vi "读取excel数据并分析.vi"() -> ()   [LabVIEW 2012]
uses:
  <vilib>/Utility/NIReport.llb/NI_report.lvclass
  <vilib>/addons/_office/excel.llb/Excel Get Data ([str]).vi
  <vilib>/addons/_office/excel.llb/Excel Easy Table (str).vi
  <vilib>/Utility/NIReport.llb/Excel/NI_Excel.lvclass
  <vilib>/addons/_office/NI_ReportGenerationToolkit.lvlib
  <vilib>/Analysis/NI_AALPro.lvlib
panel:
  in  "数据量（随具体量修改）":i32=160
  out "数组":dbl[][](array[numeric])
  out "F-格式字符串":string[][](array[string])
  in  "写入start (0, 0) 2":cluster{"row":i32, "column":i32}
  out "error out 2":errorcluster caption="错误输出"
  in  "worksheet index (0) 2":i32
  in  "template (empty) 2":path caption="写入文件位置"
  in  "error in (no error) 2":errorcluster caption="错误输入（无错误）"
  out "截距":dbl[](array[numeric])
  out "斜率":dbl[](array[numeric])
  out "子数组":dbl[](array[numeric])
  in  "读出end (-1, -1)":cluster{"row":i32, "column":i32}={"row"=-1, "column"=-1}
  out "data":string[][](array[string])
  in  "读出start (0, 0)":cluster{"start row":i32, "start column":i32}
  in  "worksheet index (0)":i32
  in  "template (empty)":path caption="读取文件位置"
  in  "error in (no error)":errorcluster caption="错误输入（无错误）"
  out "error out":errorcluster caption="错误输出"
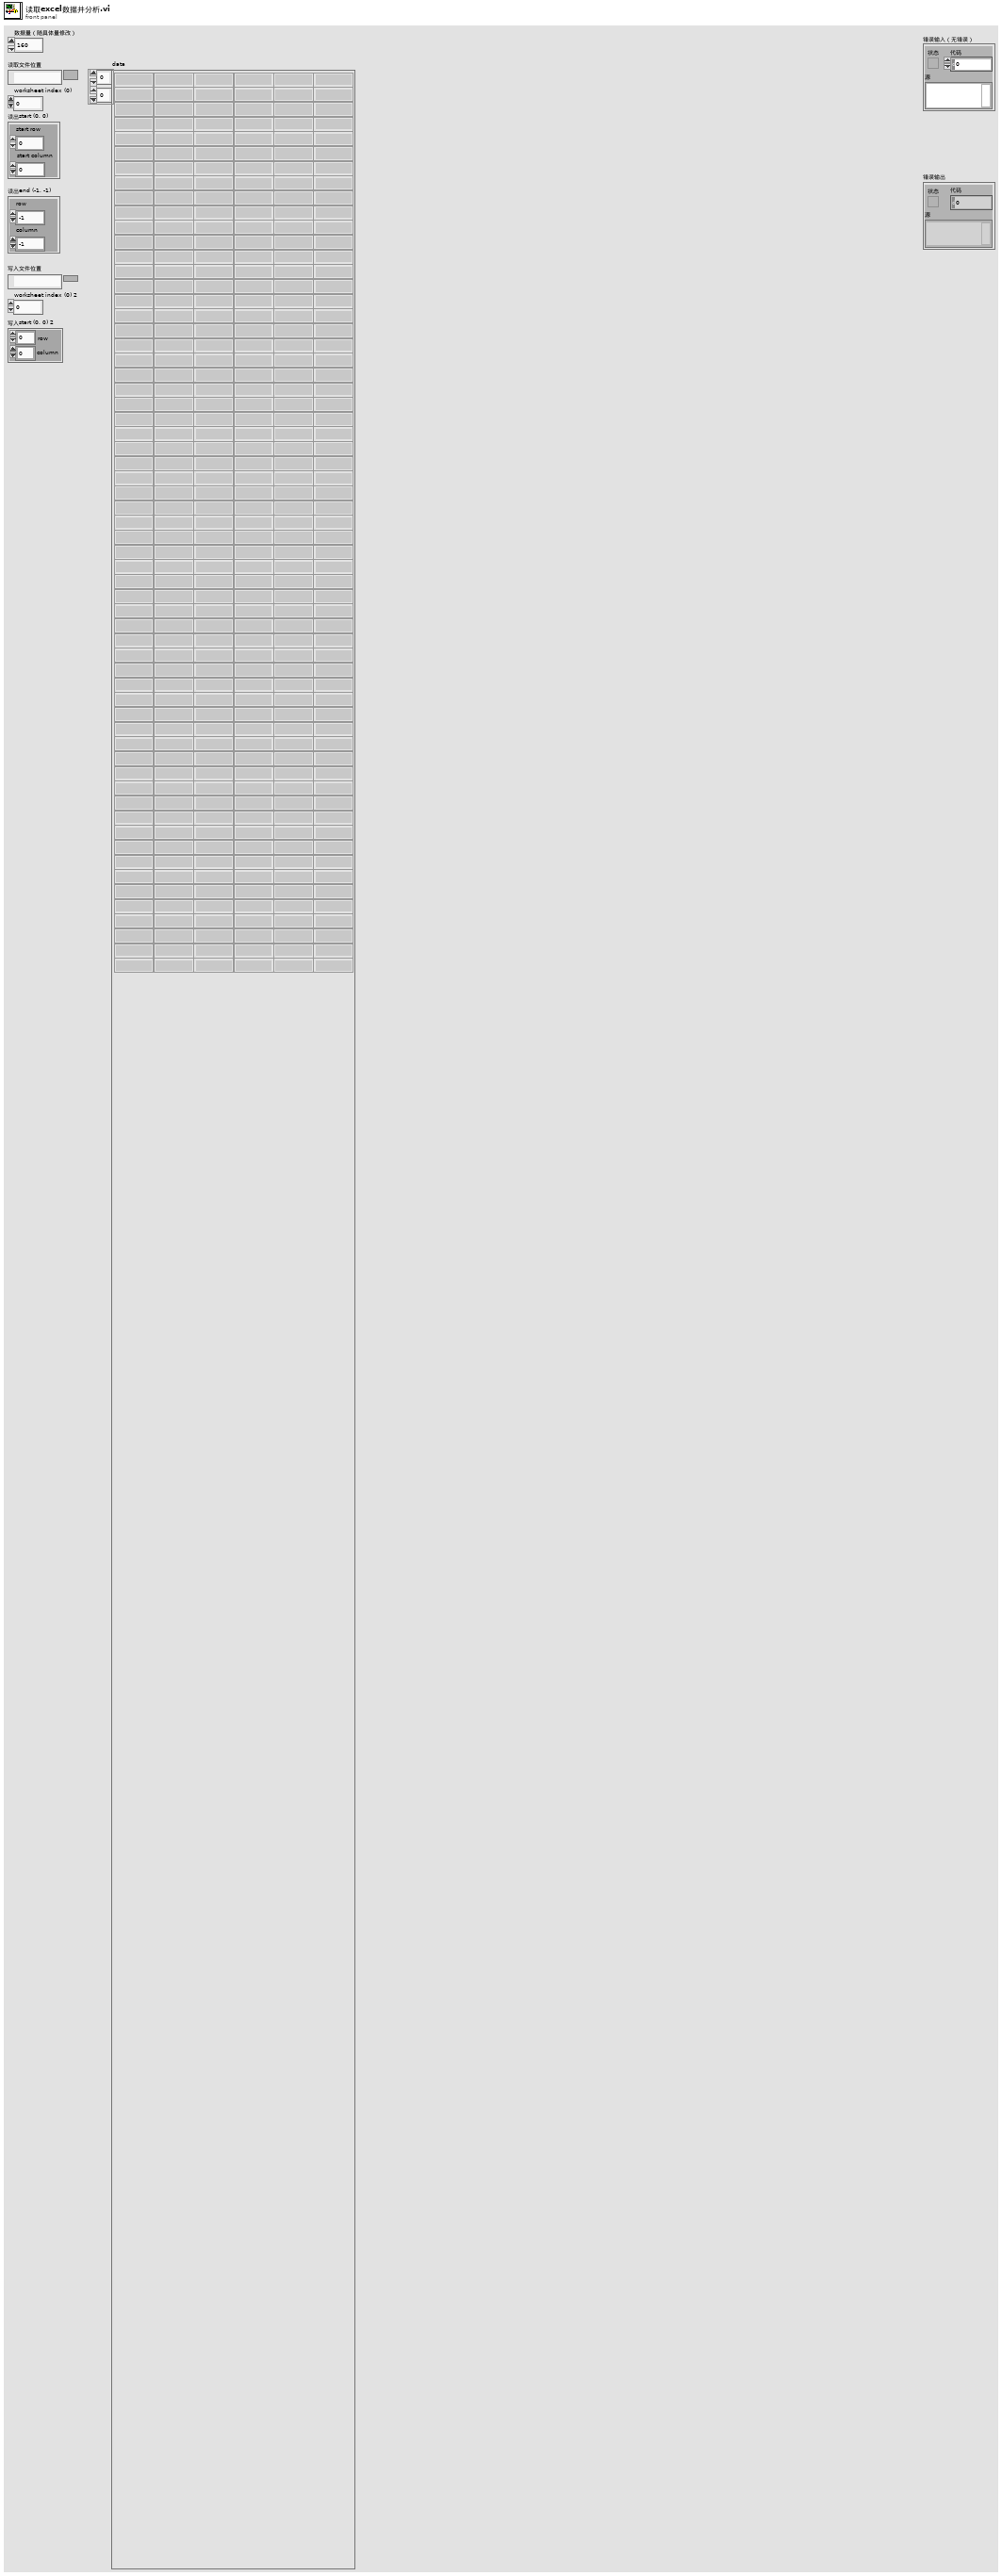
[diagram p1: front panel]
types:
  T1 = enum16{"Standard Report", "HTML", "Word", "Excel"}
  T2 = enum16{"maximized", "minimized", "normal", "no change"}
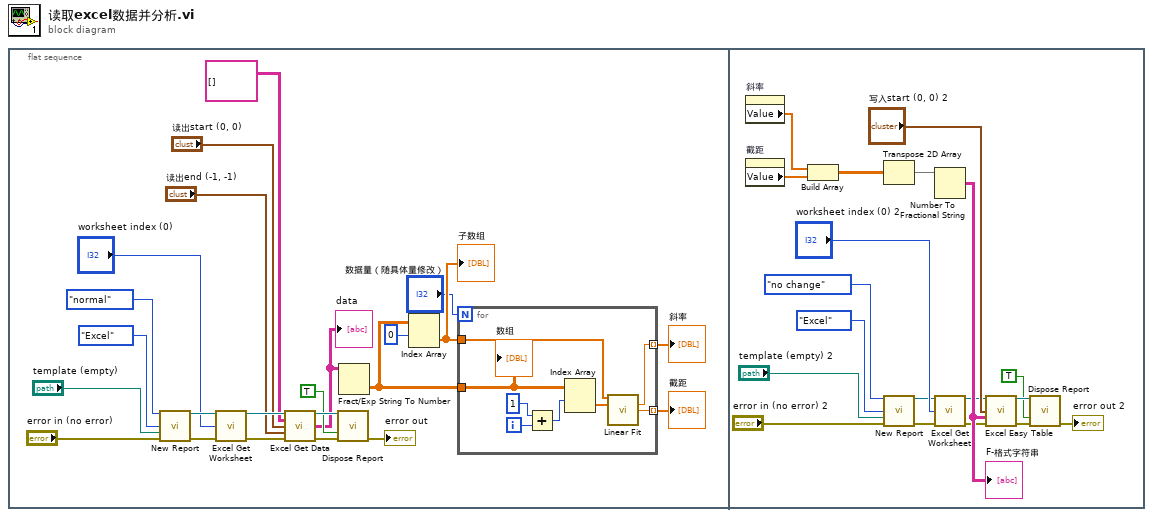
[diagram p0: block diagram]
diagram:
  n1 = flat-sequence {
    frame #0 {
      n2 = call <vilib>:"New Report.vi"("window state (normal)"=T2."normal", "report type"=T1."Excel", "template (empty)"="template (empty)", "error in (no error)"="error in (no error)") -> ("report out"=w22:refnum<class "NI_report.lvclass">, "error out"=w19:errorcluster)  [unwired: 10 in]
      n3 = call <vilib>:"Excel Get Worksheet.vi"("report in"=w22, "worksheet index (0)"="worksheet index (0)", "error in (no error)"=w19) -> ("report out"=w21:refnum<class "NI_report.lvclass">, "error out"=w18:errorcluster)  [unwired: 11 in]
      n4 = call-poly <vilib>:"Excel Get Data.vi"("report in"=w21, "data type"=string[][] [], "start (-1, -1)"="读出start (0, 0)", "end (-1, -1)"="读出end (-1, -1)", "error in (no error)"=w18) -> ("report out"=w20:refnum<class "NI_report.lvclass">, "data"=w7:string[][], "error out"=w17:errorcluster)  [unwired: 8 in]
      "data" <- w7
      n5 = call-dynamic "Dispose Report.vi"("report in"=w20, "save changes? (F)"=TRUE, "error in (no error)"=w17) -> ("error out"=→"error out":errorcluster)  [unwired: 12 in]
      n6 = Fract/Exp String To Number(string=w7) -> (number=w4:dbl[][])  [unwired: 3 in, 1 out]
      n7 = Index Array(array=w4, index (row)=0 ("索引 (行)")) -> (element=w5:dbl[])  [unwired: 1 in]
      "子数组" <- w5
      n8 = for {
        N: "数据量（随具体量修改）" -> [_]
        tunnel: w5 -> [w31]
        tunnel: w4 -> [w30]
        tunnel: [w25] -> w2 mode=indexing
        tunnel: [w24] -> w1 mode=indexing
        i -> [w29]
        n9 = Add(x=1, y=w29) -> (x+y=w27:i32)
        n10 = Index Array(array=w30, index (row)=w27) -> (element=w26:dbl[])  [unwired: 1 in]
        n11 = call <vilib>:"Linear Fit.vi"("Y"=w31, "X"=w26) -> ("slope"=w25:dbl, "intercept"=w24:dbl)  [unwired: 9 in, 3 out]
        "数组" <- w30
      }
      "斜率" <- w2
      "截距" <- w1
    }
    frame #1 {
      n12 = property on="斜率" class="Arr (严格)"() -> ("Value"=w46:dbl[])  [unwired: 2 in, 2 out]
      n13 = property on="截距" class="Arr (严格)"() -> ("Value"=w47:dbl[])  [unwired: 2 in, 2 out]
      n14 = Build Array(w46, w47) -> (w48:dbl[][])
      n15 = Transpose 2D Array(2D array=w48) -> (transposed array=w49:dbl[][])
      n16 = call <vilib>:"New Report.vi"("window state (normal)"=T2."no change", "report type"=T1."Excel", "template (empty)"="template (empty) 2", "error in (no error)"="error in (no error) 2") -> ("report out"=w33:refnum<class "NI_report.lvclass">, "error out"=w34:errorcluster)  [unwired: 10 in]
      n17 = Number To Fractional String(number=w49) -> (F-format string=w50:string[][])  [unwired: 3 in]
      "F-格式字符串" <- w50
      n18 = call <vilib>:"Excel Get Worksheet.vi"("report in"=w33, "worksheet index (0)"="worksheet index (0) 2", "error in (no error)"=w34) -> ("report out"=w41:refnum<class "NI_report.lvclass">, "error out"=w43:errorcluster)  [unwired: 11 in]
      n19 = call-poly <vilib>:"Excel Easy Table.vi"("report in"=w41, "start (0, 0)"="写入start (0, 0) 2", "text data"=w50, "error in (no error)"=w43) -> ("report out"=w42:refnum<class "NI_report.lvclass">, "error out"=w44:errorcluster)  [unwired: 7 in, 3 out]
      n20 = call-dynamic "Dispose Report.vi"("report in"=w42, "save changes? (F)"=TRUE, "error in (no error)"=w44) -> ("error out"=→"error out 2":errorcluster)  [unwired: 12 in]
    }
  }
